vi "Set Attributes Tree Data.vi"(7 "Tree ID":string, 8 "Error In":errorcluster, 9 "Attributes Values":refnum<class "Tree Data.lvclass">[](array[class]), 10 "Attributes Names":string[](array[string]), 11 "Tree Manager":T1) -> (0 "Error Out":errorcluster, 1 "Replaced?":bool[](array[boolean]), 3 "Tree Manager":T1)   [LabVIEW 2020, in "NI_VIAnCFGDataStructure.lvlib" / "Tree.lvclass"]
doc: "Set Tree Data objects as attributes of the Tree."
uses:
  <vilib>/addons/analyzer/VIAnCFGDataStructure/Tree Manager/Tree.lvclass
  <vilib>/addons/analyzer/VIAnCFGDataStructure/Tree Manager/Typedefs/Session Handle.ctl
  <vilib>/addons/analyzer/VIAnCFGDataStructure/Tree Data/Tree Data.lvclass
  <vilib>/addons/analyzer/VIAnCFGDataStructure/Tree Manager/Tree.lvclass/Tree.ctl
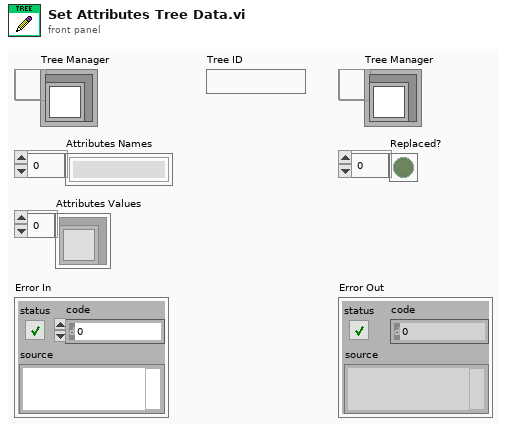
[diagram p1: front panel]
types:
  T1 = typedef "NI_VIAnCFGDataStructure.lvlib/Tree.lvclass/Session Handle.ctl" = refnum<data-value>
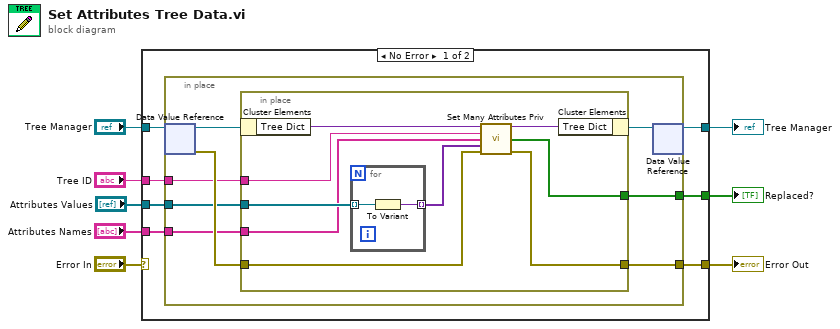
[diagram p0: block diagram]
diagram:
  n1 = case shown="No Error" "Error In" {
    selector: "Error In" -> [_ w35]
    tunnel: "Tree Manager" -> [w15 w36]
    tunnel: [w14 w36] -> w7
    tunnel: [w13 w35] -> w5
    tunnel: "Tree ID" -> [w12 _]
    tunnel: "Attributes Values" -> [w11 _]
    tunnel: "Attributes Names" -> [w10 _]
    tunnel: [w9 _] -> w2
    frame No Error {
      n2 = in-place {
        in-place-border: [w22] -> w13
        in-place-border: w12 -> [w19]
        in-place-border: w11 -> [w18]
        in-place-border: w10 -> [w17]
        in-place-border: [w16] -> w9
        n3 = in-place-dvr #1(w15) -> (w23:refnum<class "Tree.lvclass">, w20:errorcluster)
        n4 = in-place {
          in-place-border: [w28] -> w22
          in-place-border: w20 -> [w29]
          in-place-border: w19 -> [w25]
          in-place-border: w18 -> [w32]
          in-place-border: w17 -> [w24]
          in-place-border: [w27] -> w16
          n5 = in-place-cluster #2(w23) -> ("Tree Dict"=w31:variant)
          n6 = for {
            tunnel: w32 -> [w34] mode=indexing
            tunnel: [w33] -> w26 mode=indexing
            n7 = To Variant(anything=w34) -> (Variant=w33:variant)
          }
          n8 = call <vilib>:"Set Many Attributes Priv.vi"("Tree Dictionary Out"=w31, "Unique ID"=w25, "Name"=w24, "Data"=w26, "error in"=w29) -> ("Tree Dictionary Out"=w30:variant, "Replaced?"=w27:bool[], "error out"=w28:errorcluster)  [unwired: 8 in]
          n9 = in-place-cluster #2("Tree Dict"=w30) -> (w21:refnum<class "Tree.lvclass">)
        }
        n10 = in-place-dvr #1(w21) -> (w14:T1)  [unwired: 1 out]
      }
    }
    frame Error {
    }
  }
  "Tree Manager" <- w7
  "Error Out" <- w5
  "Replaced?" <- w2
